vi "initialize bank params.vi"(8 "error in (no error)":errorcluster, 9 "instrument handle in":T4, 10 "Con Chns":T3[](array[typedef]), 11 "Data Access Engine in":refnum<class "Data Access Engine.lvclass">) -> (0 "error out":errorcluster, 2 "output cluster":T1, 3 "Data Access Engine out":refnum<class "Data Access Engine.lvclass">)   [LabVIEW 2017, in "NI 272x Resistive Simulation Custom Device Engine.lvlib"]
uses:
  NI 272x Resistive Simulation Custom Device Engine.lvlib
  <instrlib>/ni272xReferenceVIs/ni272xReferenceVIs.llb/ni272x Reference.ctl
  Controls/Compiled Connect Channel.ctl
  <vilib>/NI/NIVS Inline Async API/_Data Access Engine/Data Access Engine/Data Access Engine.lvclass
  bank params.ctl
  <vilib>/NI/NIVS Inline Async API/_Data Access Engine/Data Access Engine/Types/Read.DVR.ctl
  <vilib>/NI/NIVS Inline Async API/_Data Access Engine/Access Type Classes/Read/Read.lvclass
  Globals/Names.vi
  <vilib>/NI/NIVS Inline Async API/_Data Access Engine/Data Access Engine/Methods/Read.Lookup.vi
  NI 272x Resistive Simulation Custom Device Shared.lvlib
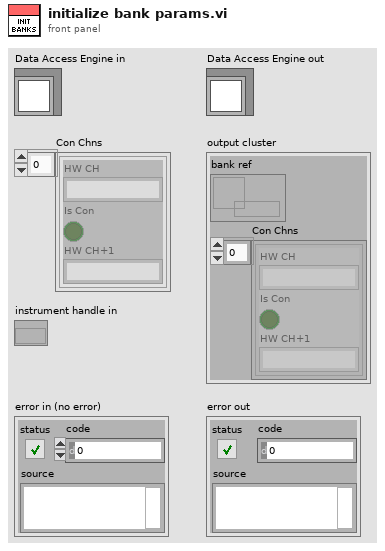
[diagram p1: front panel]
types:
  T1 = typedef "NI 272x Resistive Simulation Custom Device Engine.lvlib/bank params.ctl" = cluster{"bank ref":T2, "Con Chns":T3[]}
  T2 = typedef "Data Access Engine.lvlib/Data Access Engine.lvclass/Read.DVR.ctl" = refnum<data-value>
  T3 = typedef "NI 272x Resistive Simulation Custom Device Shared.lvlib/Compiled Connect Channel.ctl" = cluster{"HW CH":string, "Is Con":bool, "HW CH+1":string}
  T4 = typedef "ni272x Reference.ctl" = refnum<k20>
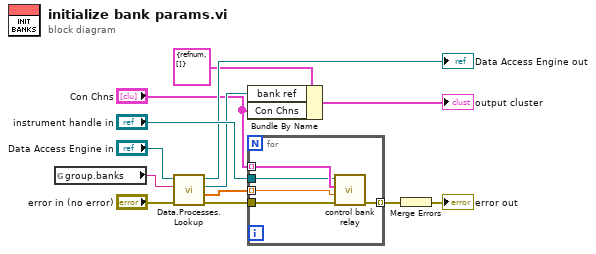
[diagram p0: block diagram]
diagram:
  n1 = global read "Names.vi" "group.banks"() -> (w7:string)
  n2 = call-poly <vilib>:"Data.Processes.Lookup.vi"("error in (no error)"="error in (no error)", "Name"=w7, "Data Access API in"="Data Access Engine in") -> ("error out"=w12:errorcluster, "Initial Values"=w8:dbl[], "Ref"=w3:T2, "Data Access API out"=→"Data Access Engine out":refnum<class "Data Access Engine.lvclass">)  [unwired: 5 in]
  n3 = Bundle By Name(cluster=T1 {"bank ref"=refnum, "Con Chns"=[]} ("bank params"), "bank ref"=w3, "Con Chns"="Con Chns") -> (→"output cluster":T1)
  n4 = for {
    tunnel: "Con Chns" -> [w18] mode=indexing
    tunnel: w8 -> [w17] mode=indexing
    tunnel: "instrument handle in" -> [w16]
    tunnel: w12 -> [w15]
    tunnel: [w14] -> w11 mode=indexing
    n5 = call "control bank relay.vi"("error in (no error)"=w15, "Channel Data Reference"=w17, "Connect Chn"=w18, "Refnum in"=w16) -> ("error out"=w14:errorcluster)  [unwired: 7 in]
  }
  n6 = Merge Errors(w11) -> (→"error out":errorcluster)
